vi "Correct Taus.vi"(4 "#_shots":i32=5, 8 "error in":errorcluster, 11 "CRDS Cell in":refnum<class "CRDS Cell.lvclass">) -> (0 "error out":errorcluster, 3 "CRDS Cell out":refnum<class "CRDS Cell.lvclass">)   [LabVIEW 2016, in "CRDS Lib.lvlib" / "CRDS Cell.lvclass"]
doc: "Correct tau values for Rayleigh scattering. \n\nIf on filter:\n* The tau and tau0 values will be the uncorrected values in seconds.\n* tau0corr will be in the Rayleigh scattering corrected value in us.\n* ext, extcorr and taucorr will be set to NaN.\n\nIf on sample:\n* Tau is the raw tau value in us.\n* taucorr will be the Rayleigh scattering corrected value in us\n* ext and extCorr will be the same value."
uses:
  CRDS Cell.lvclass
  CRDS Cell.lvclass/CRDS Cell.ctl
  Data/Cell/CRDS Cell Data.lvclass/CRDS Cell Data.ctl
  Data/Cell/Read extParam.vi
  Data/Cell/Read hkParam.vi
  General/Atmospheric/Atmospheric Constants.vi
  General/Atmospheric/Atmospheric Library.lvlib
  Data/Cell/CRDS Cell Data.lvclass
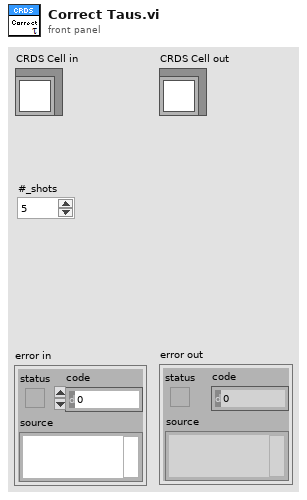
[diagram p1: front panel]
types:
  T1 = typedef "Base CRDS Lib.lvlib/calData.ctl" = cluster{"rhDilFac":sgl, "Q":sgl, "Tmean":sgl, "extDilFac":sgl, "rhCell":sgl, "P":sgl, "T":sgl}
  T2 = typedef "extparam.ctl" = cluster{"Tau":sgl, "Tau0cor":sgl, "ext":sgl, "extCorr":sgl, "stdevTau":sgl, "eTau":sgl, "taucorr":sgl, "Tau0":sgl, "max":sgl}
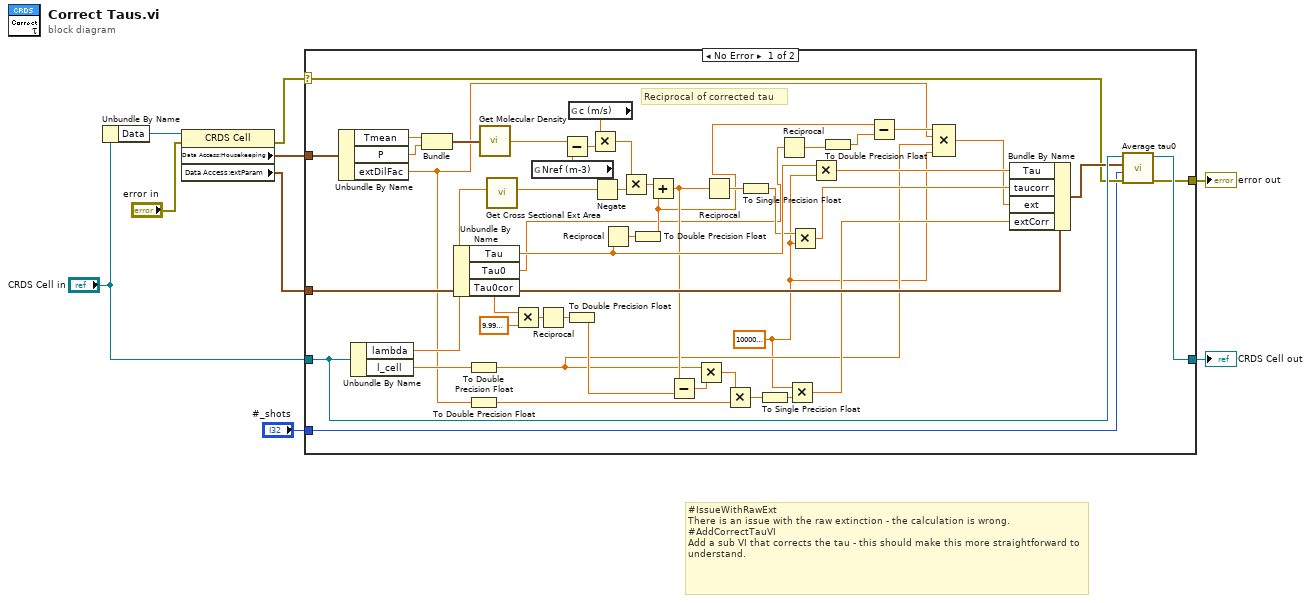
[diagram p0: block diagram]
diagram:
  # "#IssueWithRawExt\nThere is an issue with the raw extinction - the calculation is wrong.\n#AddCorrectTauVI\nAdd a sub VI that corrects the tau - this should make this more straightforward to understand."
  n1 = Unbundle By Name("CRDS Cell in") -> ("Data"=w3:refnum<class "CRDS Cell Data.lvclass">)
  n2 = property class="CRDS Cell"(reference=w3, error in="error in") -> (error out=w5:errorcluster, "Data Access:Housekeeping"=w8:T1, "Data Access:extParam"=w7:T2)  [unwired: 1 out]
  n3 = case shown="No Error" w5 {
    selector: w5 -> [w48 w59]
    tunnel: [w47 w59] -> w2
    tunnel: [w50 w58] -> w1
    tunnel: "CRDS Cell in" -> [w51 w58]
    tunnel: w8 -> [w57 _]
    tunnel: w7 -> [w55 _]
    tunnel: "#_shots" -> [w46 _]
    frame No Error {
      w10 = sgl 1000000.0
      # "Reciprocal of corrected tau"
      n4 = Unbundle By Name(w57) -> ("Tmean"=w56:sgl, "P"=w52:sgl, "extDilFac"=w13:sgl)
      n5 = Unbundle By Name(w51) -> ("lambda"=w53:dbl, "l_cell"=w54:sgl)
      n6 = Bundle("Tmean"=w56, "P"=w52) -> (w27:cluster{"Tmean":sgl, "P":sgl})  [unwired: 1 in]
      n7 = Unbundle By Name(w55) -> ("Tau"=w41:sgl, "Tau0"=w14:sgl, "Tau0cor"=w19:sgl)
      n8 = To Double Precision Float(number=w54) -> (double precision float=w12:dbl)
      n9 = To Double Precision Float(number=w13) -> (double precision float=w22:dbl)
      n10 = call "Get Molecular Density.vi"("thermoCond"=w27) -> ("M (m-3)"=w28:dbl)
      n11 = call "Get Cross Sectional Ext Area.vi"("l (nm)"=w53) -> ("CAext (m2)"=w26:dbl)  [unwired: 10 in]
      n12 = Multiply(x=w19, y=sgl 1e-06) -> (x*y=w30:sgl)
      n13 = global read "Atmospheric Constants.vi" "Nref (m-3)"() -> (w45:dbl)
      n14 = Reciprocal(x=w30) -> (1/x=w31:sgl)
      n15 = Subtract(x=w28, y=w45) -> (x-y=w40:dbl)
      n16 = To Double Precision Float(number=w31) -> (double precision float=w23:dbl)
      n17 = global read "Atmospheric Constants.vi" "c (m/s)"() -> (w39:dbl)
      n18 = Multiply(x=w39, y=w40) -> (x*y=w44:dbl)
      n19 = Negate(x=w26) -> (-x=w25:dbl)
      n20 = Reciprocal(x=w41) -> (1/x=w43:sgl)
      n21 = Multiply(x=w44, y=w25) -> (x*y=w24:dbl)
      n22 = To Double Precision Float(number=w43) -> (double precision float=w16:dbl)
      n23 = Add(x=w24, y=w16) -> (x+y=w33:dbl)
      n24 = Subtract(x=w33, y=w23) -> (x-y=w37:dbl)
      n25 = Multiply(x=w12, y=w37) -> (x*y=w34:dbl)
      n26 = Reciprocal(x=w33) -> (1/x=w32:dbl)
      n27 = Multiply(x=w34, y=w22) -> (x*y=w36:dbl)
      n28 = To Single Precision Float(number=w32) -> (single precision float=w38:sgl)
      n29 = To Single Precision Float(number=w36) -> (single precision float=w35:sgl)
      n30 = Reciprocal(x=w14) -> (1/x=w18:sgl)
      n31 = Multiply(x=w10, y=w35) -> (x*y=w20:sgl)
      n32 = Multiply(x=w38, y=w10) -> (x*y=w21:sgl)
      n33 = Multiply(x=w41, y=w10) -> (x*y=w42:sgl)
      n34 = To Double Precision Float(number=w18) -> (double precision float=w17:dbl)
      n35 = Subtract(x=w16, y=w17) -> (x-y=w15:dbl)
      n36 = Compound Arithmetic op=MULTIPLY(w15, w13, w12, w10) -> (w11:dbl)
      n37 = Bundle By Name(cluster=w55, "Tau"=w42, "taucorr"=w21, "ext"=w11, "extCorr"=w20) -> (w49:T2)
      n38 = call "Average tau0.vi"("error in"=w48, "# of shots"=w46, "extParam"=w49, "CRDS Cell in"=w51) -> ("error out"=w47:errorcluster, "CRDS Cell out"=w50:refnum<class "CRDS Cell.lvclass">)  [unwired: 6 in]
    }
    frame Error {
    }
  }
  "error out" <- w2
  "CRDS Cell out" <- w1
